vi "Log to Excel.vi"(8 "error in":errorcluster, 11 "tdms file in":refnum<k34>) -> (0 "error out":errorcluster, 2 "appended array":dbl[][][](array[numeric]), 3 "tdms file out":refnum<k34>)   [LabVIEW 2015, in "Logger.lvlib"]
uses:
  Logger.lvlib
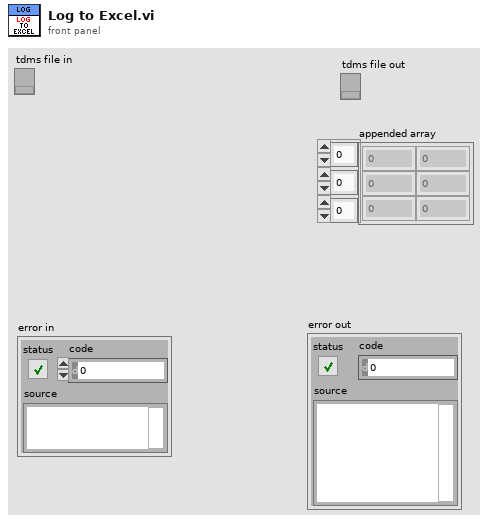
[diagram p1: front panel]
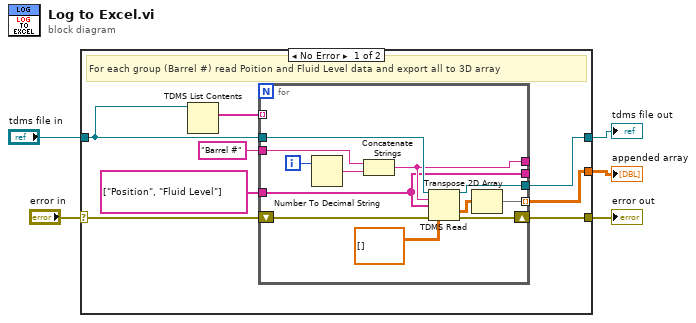
[diagram p0: block diagram]
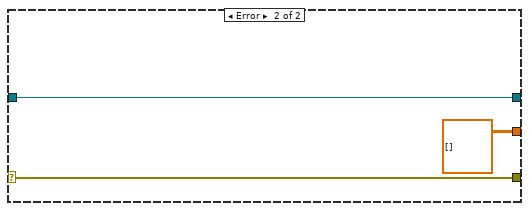
[diagram p2: hidden frame]
diagram:
  n1 = case shown="No Error" "error in" {
    selector: "error in" -> [w6 w28]
    tunnel: [w12 dbl[][][] []] -> w5
    tunnel: [w11 w28] -> w4
    tunnel: [w9 w27] -> w3
    tunnel: "tdms file in" -> [w8 w27]
    frame No Error {
      # "For each group (Barrel #) read Poition and Fluid Level data and export all to 3D array"
      n2 = TDMS List Contents(7:w8) -> (2:w7:string[])  [unwired: 2 in, 3 out]
      n3 = for {
        tunnel: w8 -> [w25]
        tunnel: string[] ["Position", "Fluid Level"] -> [w16]
        tunnel: "Barrel #" -> [w22]
        tunnel: [w14] -> w12 mode=indexing
        tunnel: [w18] -> w9
        shift-right: [w19] -> w11
        shift-left: w6 -> [w24]
        tunnel: [w16] -> _
        tunnel: [w17] -> _
        tunnel: w7 -> [_] mode=indexing
        i -> [w20]
        n4 = Number To Decimal String(number=w20) -> (decimal integer string=w21:string)  [unwired: 1 in]
        n5 = Concatenate Strings(w22, w21) -> (w17:string)
        n6 = TDMS Read(0:w25, 5:w17, 7:w16, 11:w24, 12:dbl[][] [] ("appended array")) -> (4:w18:refnum<k34>, 10:w15:dbl[][], 15:w19:errorcluster)  [unwired: 3 in, 3 out]
        n7 = Transpose 2D Array(2D array=w15) -> (transposed array=w14:dbl[][])
      }
    }
    frame Error {
    }
  }
  "error out" <- w4
  "appended array" <- w5
  "tdms file out" <- w3
